vi "Command Deliver Gear.vi"(2 "Robot System Functions In":T1, 3 "Startup":bool, 4 "String Parameter":string, 5 "Cmd Parameter 3":dbl, 6 "Speed at which the Gear Delivers":dbl, 7 "Time To Run":dbl) -> (0 "Robot System Functions Out":T1, 1 "Completed":bool)   [LabVIEW 2016]
uses:
  Subsystems/All Robot Commands.ctl
  Subsystems/Drive and Climb SS/Drive + Climb Commands 2017.ctl
  Subsystems/Gear Delivery SS/Gear Delivery Commands.ctl
  Subsystems/Conveyor and Shooter SS/Conveyor and Shooter Commands.ctl
  Subsystems/Ball Intake SS/Ball Intake Commands.ctl
  Command Execution State.ctl
panel:
  # "Sample robot\ncontrol output.\nReplace with \nactual teleop \ncontrol signal \nstructure."
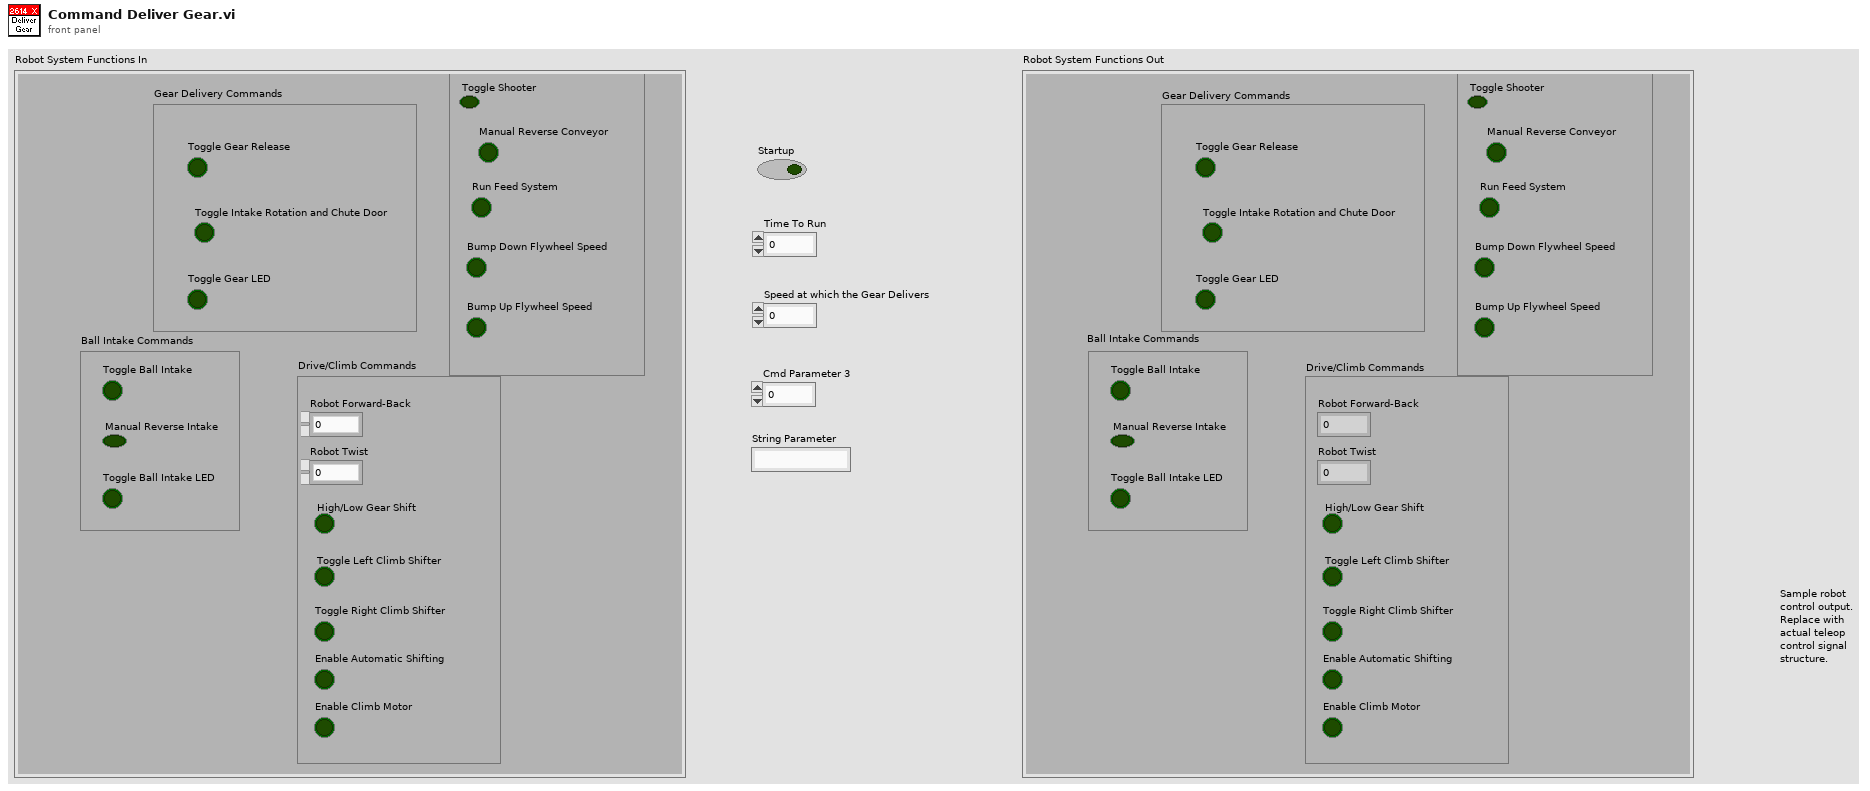
[diagram p1: front panel]
types:
  T1 = typedef "All Robot Commands.ctl" = cluster{"Drive/Climb Commands":T2, "Gear Delivery Commands":T3, "Shooter and Conveyor Commands":T4, "Ball Intake Commands":T5}
  T2 = typedef "Drive + Climb Commands 2017.ctl" = cluster{"Robot Forward-Back":dbl, "Robot Twist":dbl, "High/Low Gear Shift":bool, "Toggle Left Climb Shifter":bool, "Toggle Right Climb Shifter":bool, "Enable Automatic Shifting":bool, "Enable Climb Motor ":bool}
  T3 = typedef "Gear Delivery Commands.ctl" = cluster{"Toggle Gear Release":bool, "Toggle Intake Rotation and Chute Door":bool, "Toggle Gear LED":bool}
  T4 = typedef "Conveyor and Shooter Commands.ctl" = cluster{"Toggle Shooter":bool, "Manual Reverse Conveyor":bool, "Run Feed System":bool, "Bump Down Flywheel Speed":bool, "Bump Up Flywheel Speed":bool}
  T5 = typedef "Ball Intake Commands.ctl" = cluster{"Toggle Ball Intake":bool, "Manual Reverse Intake":bool, "Toggle Ball Intake LED":bool}
  T6 = typedef "Command Execution State.ctl" = enum16{"Initialize", "Execute", "Finish"}
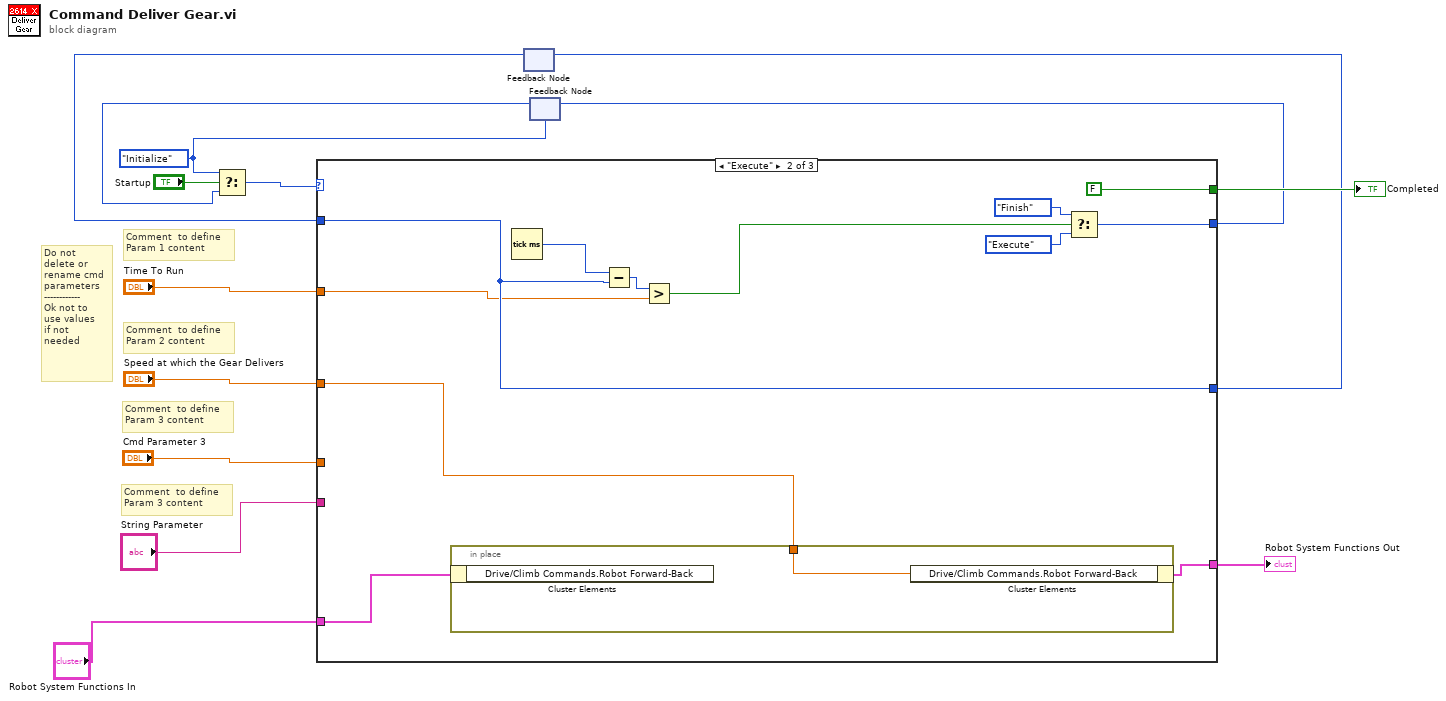
[diagram p0: block diagram]
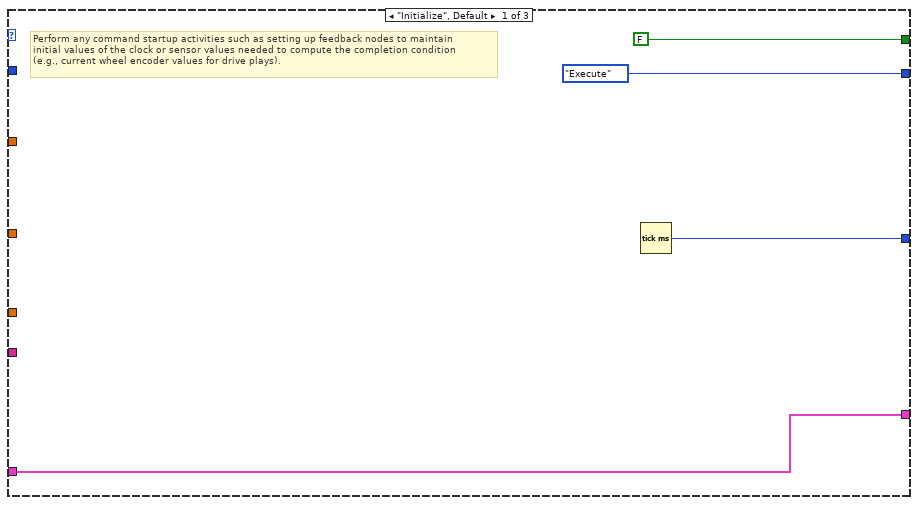
[diagram p2: hidden frame]
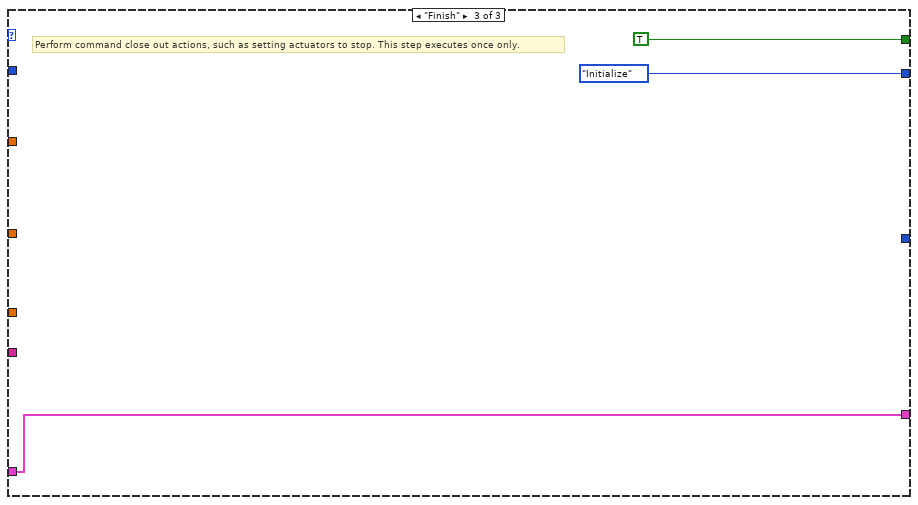
[diagram p3: hidden frame]
diagram:
  w9 = Command_Execution_State."Initialize" ("Play State")
  # "Comment  to define\nParam 3 content"
  # "Comment  to define\nParam 3 content"
  # "Do not \ndelete or\nrename cmd\nparameters\n------------\nOk not to \nuse values\nif not \nneeded"
  # "Comment  to define\nParam 2 content"
  # "Comment  to define\nParam 1 content"
  n1 = feedback #1() -> (w1:u32)  [unwired: 1 in]
  n2 = feedback #2(w9) -> (w10:T6)
  n3 = Select(t=w9, s="Startup", f=w10) -> (s? t:f=w14:T6)
  n4 = case shown="\"Execute\"" w14 {
    tunnel: [FALSE FALSE TRUE] -> w12
    tunnel: [Command_Execution_State."Execute" ("Play State") w28 Command_Execution_State."Initialize" ("f")] -> w11
    tunnel: "Time To Run" -> [_ w22 _]
    tunnel: "Speed at which the Gear Delivers" -> [_ w20 _]
    tunnel: [w16 w19 w32] -> w6
    tunnel: "Robot System Functions In" -> [w16 w26 w32]
    tunnel: "Cmd Parameter 3" -> [_ _ _]
    tunnel: "String Parameter" -> [_ _ _]
    tunnel: [w15 w24 _] -> w2
    tunnel: w1 -> [_ w24 _]
    frame "Initialize", Default {
      # "Perform any command startup activities such as setting up feedback nodes to maintain \ninitial values of the clock or sensor values needed to compute the completion condition\n(e.g., current wheel encoder values for drive plays)."
      n5 = Tick Count (ms)() -> (millisecond timer value=w15:u32)
    }
    frame "Execute" {
      n6 = in-place {
        in-place-border: w20 -> [w31]
        n7 = in-place-cluster #3(w26) -> ()  [unwired: 1 out]
        n8 = in-place-cluster #3("Drive/Climb Commands.Robot Forward-Back"=w31) -> (w19:T1)
      }
      n9 = Tick Count (ms)() -> (millisecond timer value=w25:u32)
      n10 = Subtract(x=w25, y=w24) -> (x-y=w23:u32)
      n11 = Greater?(x=w23, y=w22) -> (0:w21:bool)
      n12 = Select(t=Command_Execution_State."Finish" ("Play State"), s=w21, f=Command_Execution_State."Execute") -> (s? t:f=w28:T6)
    }
    frame "Finish" {
      # "Perform command close out actions, such as setting actuators to stop. This step executes once only."
    }
  }
  "Completed" <- w12
  "Robot System Functions Out" <- w6
  n13 = feedback-in #1(w2) -> ()
  n14 = feedback-in #2(w11) -> ()
